vi "Calc.vi"(8 "error in (no error)":errorcluster, 10 "ArrayOfWVFMs":waveform(dbl)[](array[waveform]), 11 "Mean in":refnum<class "Mean.lvclass">) -> (0 "error out":errorcluster, 2 "Results":string[](array[string]), 3 "Mean out":refnum<class "Mean.lvclass">)   [LabVIEW 2015, in "MeanLib.lvlib" / "Mean.lvclass"]
uses:
  Mean.lvclass
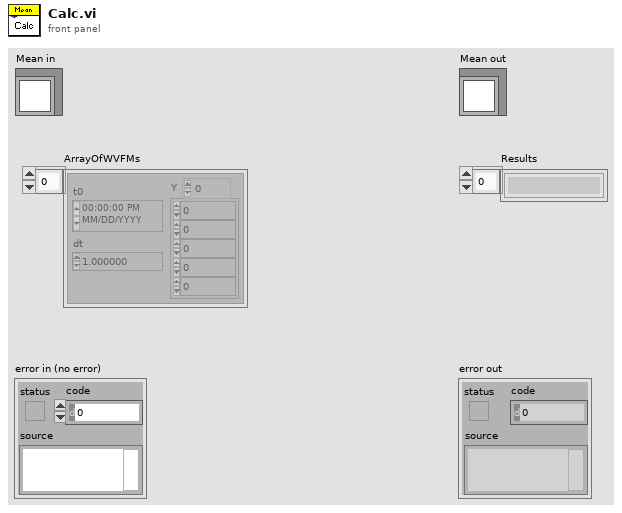
[diagram p1: front panel]
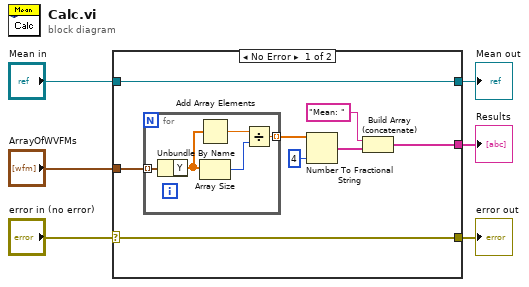
[diagram p0: block diagram]
diagram:
  n1 = case shown="No Error" "error in (no error)" {
    selector: "error in (no error)" -> [w14 _]
    tunnel: [w7 _] -> w6
    tunnel: [w14 _] -> w4
    tunnel: "ArrayOfWVFMs" -> [w13 _]
    tunnel: "Mean in" -> [w12 w20]
    tunnel: [w12 w20] -> w1
    frame No Error {
      n2 = for {
        tunnel: w13 -> [w19] mode=indexing
        tunnel: [w15] -> w11 mode=indexing
        n3 = Unbundle By Name(w19) -> ("Y"=w16:dbl[])
        n4 = Add Array Elements(numeric array=w16) -> (sum=w18:dbl)
        n5 = Array Size(array=w16) -> (size(s)=w17:i32)
        n6 = Divide(x=w18, y=w17) -> (x/y=w15:dbl)
      }
      n7 = Number To Fractional String(number=w11, precision (6)=i16 4) -> (F-format string=w8:string[])  [unwired: 2 in]
      n8 = Build Array (concatenate)("Mean: ", w8) -> (w7:string[])
    }
    frame Error {
    }
  }
  "error out" <- w4
  "Mean out" <- w1
  "Results" <- w6
